vi "Exclusion Data To Tree.vi"(6 "Test Hierarchy":T1[](array[typedef]), 7 "Owning Tree":string, 8 "error in":errorcluster, 9 "Config File":path, 10 "Exclusion Data":T3[](array[typedef]), 11 "Tree Manager in":T2) -> (0 "error out":errorcluster, 3 "Tree Manager out":T2)   [LabVIEW 2020]
uses:
  <vilib>/addons/analyzer/_analyzerctrls.llb/VIAnCtl Exclusion Data.ctl
  <vilib>/addons/analyzer/VIAnCFGDataStructure/Tree Manager/Typedefs/Session Handle.ctl
  <vilib>/addons/analyzer/VIAnCFGDataStructure/Tree Manager/Tree.lvclass
  <vilib>/addons/analyzer/_analyzerctrls.llb/VIAnCtl TreeHierarchy.ctl
  <vilib>/addons/analyzer/VIAnCFGDataStructure/Data Types/Path/Path.lvclass/Path.ctl
  <vilib>/addons/analyzer/VIAnCFGDataStructure/Data Types/String Array/1D String.lvclass/1D String.ctl
  <vilib>/addons/analyzer/VIAnCFGDataStructure/Data Types/String Array/To 1D String Tree Data.vi
  <vilib>/addons/analyzer/VIAnCFGDataStructure/Data Types/Path/To Path Tree Data.vi
  <vilib>/addons/analyzer/VIAnCFGDataStructure/Data Types/String Array/1D String.lvclass
  e:/builds/penguin/labview/branches/2020/dev/dist/vi.lib/addons/analyzer/VIAnCFGDataStructure/Tree Data/Tree Data.lvclass
  <vilib>/addons/analyzer/VIAnCFGDataStructure/Data Types/Path/Path.lvclass
  <vilib>/addons/analyzer/_vianuishared.llb/VIAnUI CFG File Info Global.vi
  <vilib>/addons/analyzer/VIAnCFGDataStructure/Tree Manager/API/Set Attribute Tree Data.vi
  e:/builds/penguin/labview/branches/2020/dev/dist/vi.lib/addons/analyzer/VIAnCFGDataStructure/Data Types/Path/Path.lvclass
  e:/builds/penguin/labview/branches/2020/dev/dist/vi.lib/addons/analyzer/VIAnCFGDataStructure/Data Types/String Array/1D String.lvclass
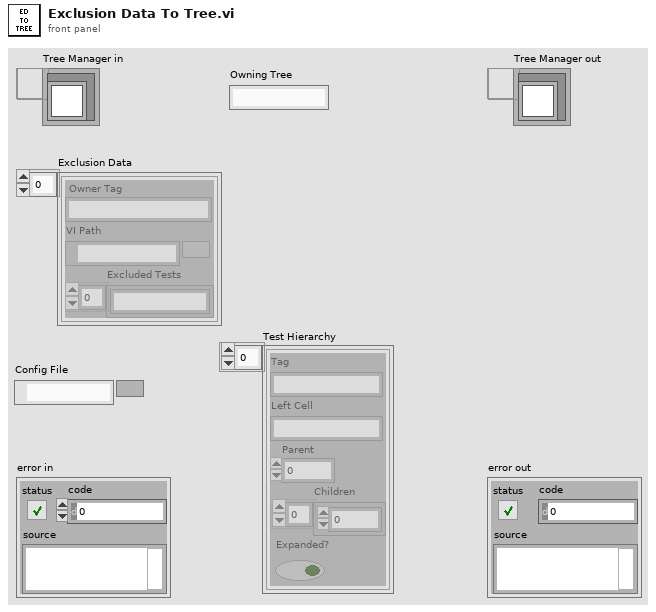
[diagram p1: front panel]
types:
  T1 = typedef "VIAnCtl TreeHierarchy.ctl" = cluster{"Tag":string, "Left Cell":string, "Parent":i32, "Children":i32[], "Expanded?":bool}
  T2 = typedef "NI_VIAnCFGDataStructure.lvlib/Tree.lvclass/Session Handle.ctl" = refnum<data-value>
  T3 = typedef "VIAnCtl Exclusion Data.ctl" = cluster{"Owner Tag":string, "VI Path":path, "Excluded Tests":string[]}
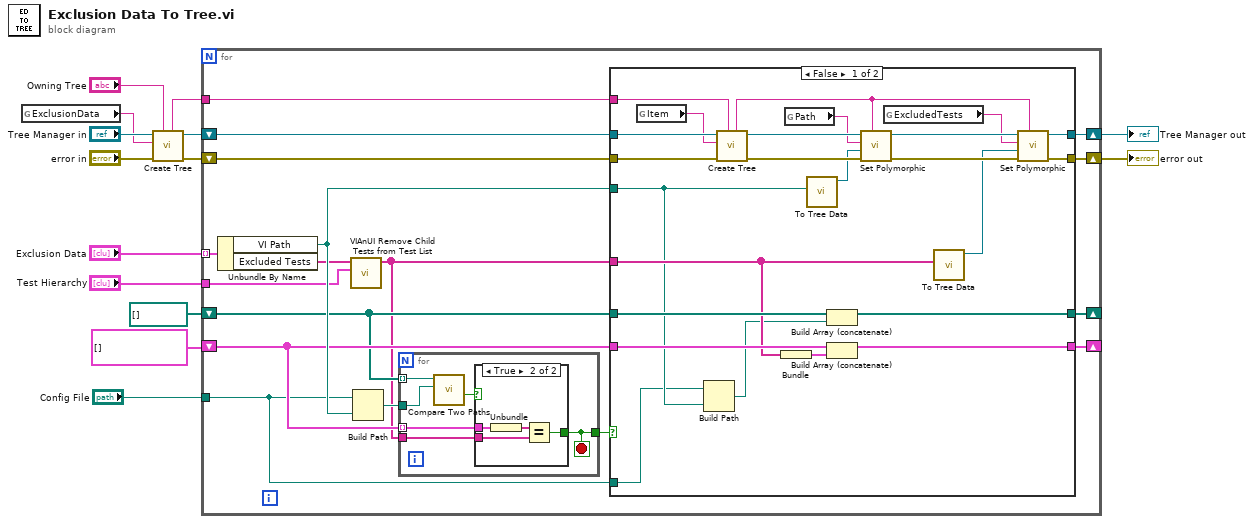
[diagram p0: block diagram]
diagram:
  n1 = global read "VIAnUI CFG File Info Global.vi" "ExclusionData"() -> (w6:string)
  n2 = call <vilib>:"Create Tree.vi"("Parent ID (empty)"="Owning Tree", "Error In"="error in", "Name"=w6, "Tree Manager"="Tree Manager in") -> ("Error Out"=w10:errorcluster, "Tree Manager"=w11:T2, "Unique ID"=w9:string)  [unwired: 5 in]
  n3 = for {
    tunnel: "Exclusion Data" -> [w31] mode=indexing
    shift-right: [w27] -> w7
    shift-left: w11 -> [w30]
    shift-right: [w26] -> w14
    shift-left: w10 -> [w29]
    tunnel: w9 -> [w28]
    shift-right: [w25] -> _
    shift-left: path[] [] -> [w20]
    shift-right: [w24] -> _
    shift-left: cluster{string[]}[] [] -> [w21]
    tunnel: "Config File" -> [w18]
    tunnel: "Test Hierarchy" -> [w15]
    n4 = Unbundle By Name(w31) -> ("VI Path"=w23:path, "Excluded Tests"=w17:string[])
    n5 = call <vilib>:"VIAnUI Remove Child Tests from Test List.vi"("Test Hierarchy"=w15, "Tests in"=w17) -> ("Tests out"=w16:string[])  [unwired: 9 in]
    n6 = Build Path(base path=w18, name or relative path=w23) -> (appended path=w22:path)
    n7 = for {
      tunnel: w22 -> [w36]
      tunnel: w21 -> [w34] mode=indexing
      tunnel: w20 -> [w37] mode=indexing
      tunnel: w16 -> [w33]
      tunnel: [w32] -> w19
      stop <- w32 stop-if-true
      n8 = call <vilib>:"Compare Two Paths.vi"("Path 2"=w36, "Path 1"=w37) -> ("Path 2 Relative to Path 1?"=w35:bool)  [unwired: 6 in, 3 out]
      n9 = case shown="True" w35 {
        selector: w35 -> [w38 _]
        tunnel: w34 -> [_ w42]
        tunnel: w33 -> [_ w40]
        tunnel: [w38 w39] -> w32
        frame False {
        }
        frame True {
          n10 = Unbundle(w42) -> (w41:string[])
          n11 = Equal?(x=w41, y=w40) -> (x = y?=w39:bool)
        }
      }
    }
    n12 = case shown="False" w19 {
      tunnel: w30 -> [w66 w70]
      tunnel: w29 -> [w65 w69]
      tunnel: w28 -> [w64 _]
      tunnel: [w57 w70] -> w27
      tunnel: [w56 w69] -> w26
      tunnel: w23 -> [w44 _]
      tunnel: w16 -> [w47 _]
      tunnel: w20 -> [w51 w68]
      tunnel: [w49 w68] -> w25
      tunnel: [w48 w67] -> w24
      tunnel: w21 -> [w50 w67]
      tunnel: w18 -> [w43 _]
      frame False {
        n13 = global read "VIAnUI CFG File Info Global.vi" "Item"() -> (w54:string)
        n14 = Build Path(base path=w43, name or relative path=w44) -> (appended path=w45:path)
        n15 = call <vilib>:"Create Tree.vi"("Parent ID (empty)"=w64, "Error In"=w65, "Name"=w54, "Tree Manager"=w66) -> ("Error Out"=w62:errorcluster, "Tree Manager"=w63:T2, "Unique ID"=w60:string)  [unwired: 5 in]
        n16 = Bundle("Tests out"=w47) -> (w46:cluster{"Tests out":string[]})  [unwired: 1 in]
        n17 = global read "VIAnUI CFG File Info Global.vi" "Path"() -> (w53:string)
        n18 = call-poly <vilib>:"To Tree Data.vi"("Path"=w44) -> ("Path Tree Data"=w55:refnum<class "Path.lvclass">)  [unwired: 10 in]
        n19 = Build Array (concatenate)(w51, w45) -> (w49:path[])
        n20 = Build Array (concatenate)(w50, w46) -> (w48:cluster{"Tests out":string[]}[])
        n21 = call-poly <vilib>:"Set Polymorphic.vi"("Tree ID"=w60, "Error In"=w62, "Attribute Value"=w55, "Attribute Name"=w53, "Tree Manager"=w63) -> ("Error Out"=w59:errorcluster, "Tree Manager"=w61:T2)  [unwired: 4 in, 1 out]
        n22 = global read "VIAnUI CFG File Info Global.vi" "ExcludedTests"() -> (w52:string)
        n23 = call-poly <vilib>:"To Tree Data.vi"("1D String"=w47) -> ("1D String Tree Data"=w58:refnum<class "1D String.lvclass">)  [unwired: 10 in]
        n24 = call-poly <vilib>:"Set Polymorphic.vi"("Tree ID"=w60, "Error In"=w59, "Attribute Value"=w58, "Attribute Name"=w52, "Tree Manager"=w61) -> ("Error Out"=w56:errorcluster, "Tree Manager"=w57:T2)  [unwired: 4 in, 1 out]
      }
      frame True {
        # "This path already has a parent in the list that shares the same 'Excluded Tests' setting. No need to add it to the XML."
      }
    }
  }
  "error out" <- w14
  "Tree Manager out" <- w7
